vi "Save All VIs.vi"(8 "error in (no error)":errorcluster, 11 "Model in":refnum<class "Model.lvclass">) -> (0 "error out":errorcluster, 3 "Model out":refnum<class "Model.lvclass">)   [LabVIEW 2018, in "Model.lvlib" / "Model.lvclass"]
uses:
  Model.lvclass
  Model.lvclass/Model.ctl
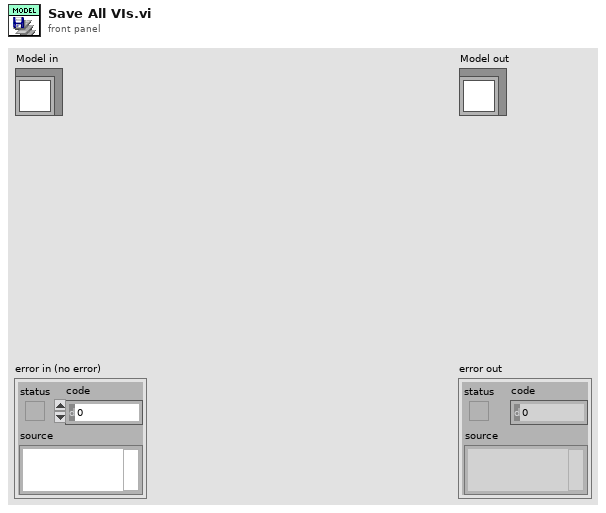
[diagram p1: front panel]
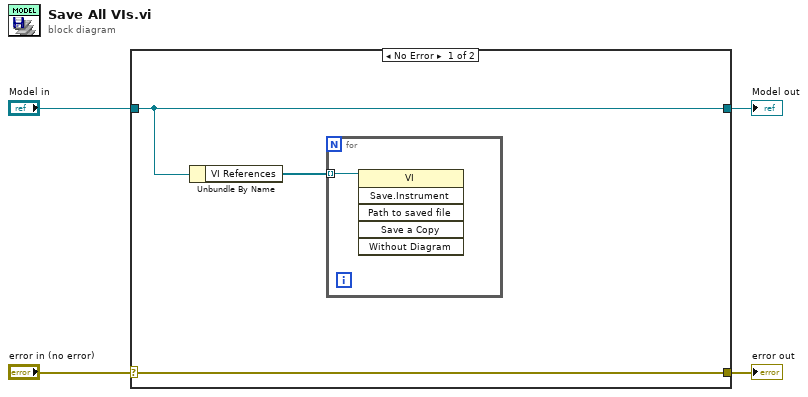
[diagram p0: block diagram]
diagram:
  n1 = case shown="No Error" "error in (no error)" {
    selector: "error in (no error)" -> [w7 w10]
    tunnel: [w7 w10] -> w3
    tunnel: [w6 w9] -> w1
    tunnel: "Model in" -> [w6 w9]
    frame No Error {
      n2 = Unbundle By Name(w6) -> ("VI References"=w5:refnum<vi>[])
      n3 = for {
        tunnel: w5 -> [w8] mode=indexing
        n4 = invoke class="VI" method="Save.Instrument"(reference=w8) -> ()  [unwired: 5 in, 6 out]
      }
    }
    frame Error {
    }
  }
  "error out" <- w3
  "Model out" <- w1
